vi "WriteModeDM_STED.vi"(5 "ClearV":bool, 7 "Flat On":bool, 9 "Amplitudes":dbl[](array[numeric]), 10 "Modes":i32[](array[numeric])) -> (0 "V Map":dbl[](array[numeric]), 3 "Voltage Map":dbl[][](array[numeric]))   [LabVIEW 2014]
uses:
  <vilib>/Analysis/baseanly.llb/A x Vector.vi
  <vilib>/Analysis/NI_AALBase.lvlib
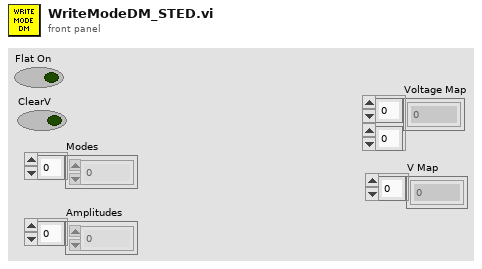
[diagram p1: front panel]
types:
  T1 = typedef "NI_Matrix.lvlib/RealMatrix.ctl" = dbl[][]
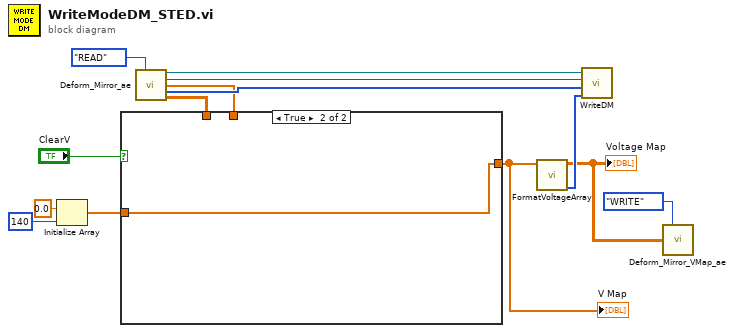
[diagram p0: block diagram]
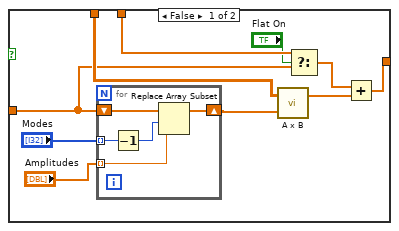
[diagram p2: hidden frame]
diagram:
  n1 = Initialize Array(0.0 ("element"), 140 ("dimension size")) -> (w5:dbl[])
  n2 = call "Deform_Mirror_ae.vi"("Enum"=enum16{"WRITE", "READ"}."READ") -> ("Refnum Out"=w9:refnum<k7>, "IDs Out"=w7:i32, "Flat Files Out"=w6:dbl[], "Multi Map Data Out"=w8:i32[], "Mode Matrix Out"=w10:T1)  [unwired: 10 in]
  n3 = case shown="True" "ClearV" {
    tunnel: w10 -> [w21 _]
    tunnel: w6 -> [w20 _]
    tunnel: w5 -> [w19 w30]
    tunnel: [w15 w30] -> w4
    frame False {
      n4 = for {
        tunnel: "Modes" -> [w28] mode=indexing
        tunnel: "Amplitudes" -> [w26] mode=indexing
        shift-right: [w25] -> w22
        shift-left: w19 -> [w29]
        n5 = Decrement(x=w28) -> (x-1=w27:i32)
        n6 = Replace Array Subset(array=w29, new element=w26, index=w27) -> (w25:dbl[])
      }
      n7 = call-poly <vilib>:"A x B.vi"("Vector"=w22, "A"=w21) -> ("A x Vector"=w18:dbl[])  [unwired: 1 out]
      n8 = Select(t=w20, s="Flat On", f=w19) -> (s? t:f=w17:dbl[])
      n9 = Add ("Add.vi")(x=w17, y=w18) -> (x+y=w15:dbl[])
    }
    frame True {
    }
  }
  "V Map" <- w4
  n10 = call "FormatVoltageArray.vi"("Array in"=w4) -> ("Mirror Array"=w11:u16[], "Voltage Map"=w2:dbl[][])  [unwired: 9 in]
  "Voltage Map" <- w2
  n11 = call "WriteDM.vi"("reference in"=w9, "nDevId"=w7, "MultiDM  Mapping"=w8, "Voltage Array in"=w11) -> ()  [unwired: 2 in, 2 out]
  n12 = call "Deform_Mirror_VMap_ae.vi"("Action"=enum16{"WRITE", "READ"}."WRITE", "V Map In"=w2) -> ()  [unwired: 13 in, 1 out]
